vi "Config Display.vi"(0 "VISA resource name":refnum<visa-resource-name>, 1 "Display Brightness (2: 75%)":u16(ring)=2 items=["25%", "50%", "75%", "100%"], 2 "Number of Locations (1)":dbl=1.0 min=1.0 max=8.0 step=1.0, 5 "Location (1)":dbl=1.0 min=1.0 max=8.0 step=1.0, 7 "Channel (1)":i32=1 min=0 max=16 step=1, 9 "Source (0: Kelvin)":u16(ring) items=["Kelvin", "Ohms", "Linear Data", "Min Data", "Max Data"], 11 "error in (no error)":errorcluster, 12 "Resolution (4)":i32=4 min=4 max=6 step=1) -> (4 "VISA resource name out":refnum<visa-resource-name>, 15 "error out":errorcluster)   [LabVIEW 2012, in "Lake Shore Cryotronics 370.lvlib"]
doc: "This VI Configures the parameters of the front panel display."
uses:
  <instrlib>/Lake Shore Cryotronics 370/Lake Shore Cryotronics 370.lvlib
panel:
  # "Displayed Location Parameters"
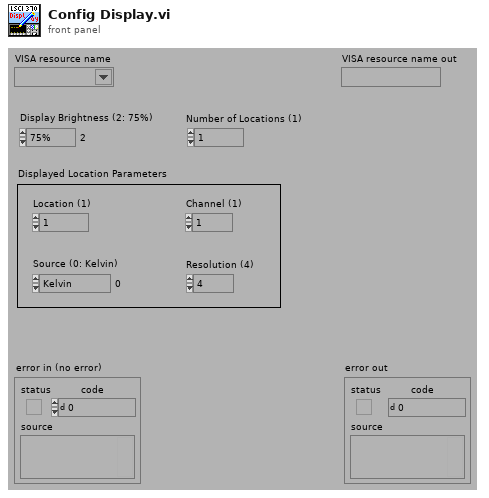
[diagram p1: front panel]
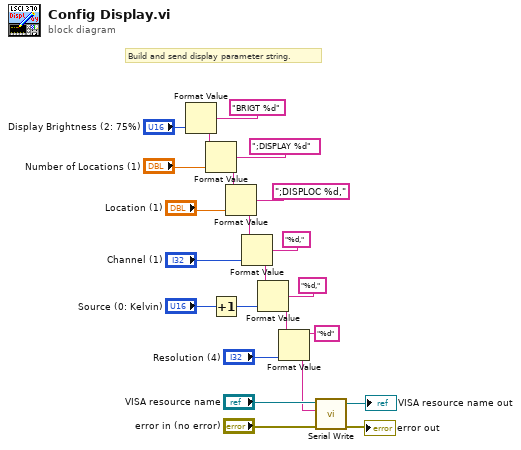
[diagram p0: block diagram]
diagram:
  # "Build and send display parameter string."
  n1 = Format Value(format string="BRIGT %d", value (0)="Display Brightness (2: 75%)") -> (output string=w8:string)  [unwired: 1 in]
  n2 = Format Value(string ("")=w8, format string=";DISPLAY %d", value (0)="Number of Locations (1)") -> (output string=w7:string)
  n3 = Increment(x="Source (0: Kelvin)") -> (x+1=w22:u16)
  n4 = Format Value(string ("")=w7, format string=";DISPLOC %d,", value (0)="Location (1)") -> (output string=w11:string)
  n5 = Format Value(string ("")=w11, format string="%d,", value (0)="Channel (1)") -> (output string=w10:string)
  n6 = Format Value(string ("")=w10, format string="%d,", value (0)=w22) -> (output string=w4:string)
  n7 = Format Value(string ("")=w4, format string="%d", value (0)="Resolution (4)") -> (output string=w3:string)
  n8 = call <instrlib>:"Serial Write.vi"("error in (no error)"="error in (no error)", "Write Buffer (\"\")"=w3, "VISA resource name"="VISA resource name") -> ("error out"=→"error out":errorcluster, "VISA resource name out"=→"VISA resource name out":refnum<visa-resource-name>)  [unwired: 6 in, 1 out]
